vi "set Line Colour.vi"(10 "Line Colour":u32(colorbox), 11 "Scene in":refnum<class "Scene.lvclass">) -> (3 "Scene out":refnum<class "Scene.lvclass">)   [LabVIEW 2020, in "Scene.lvclass"]
uses:
  Scene.lvclass
  Scene.lvclass/Scene.ctl
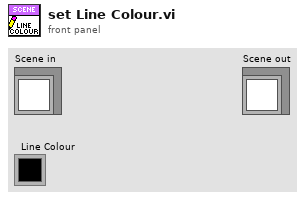
[diagram p1: front panel]
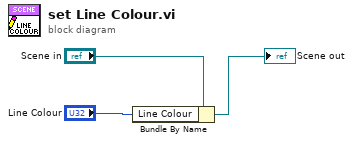
[diagram p0: block diagram]
diagram:
  n1 = Bundle By Name(cluster="Scene in", "Line Colour"="Line Colour") -> (→"Scene out":refnum<class "Scene.lvclass">)
